vi "Fetch_DMM2831E .vi"(3 "error in (no error)":errorcluster, 5 "VISA resource name":refnum<visa-resource-name>) -> (0 "error out":errorcluster, 1 "Measurement":dbl, 2 "VISA resource name out":refnum<visa-resource-name>)   [LabVIEW 2023]
uses:
  <instrlib>/BK Precision 5491B/BK Precision 5491B.lvlib
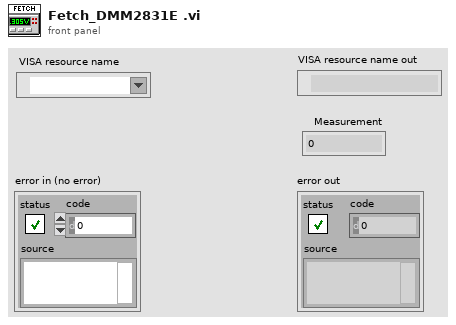
[diagram p1: front panel]
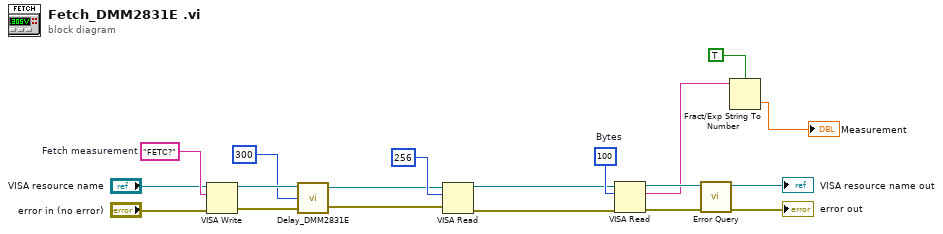
[diagram p0: block diagram]
diagram:
  w14 = "FETC?"  # Fetch measurement
  w19 = u32 100  # Bytes
  n1 = VISA Write(VISA resource name="VISA resource name", write buffer=w14, error in (no error)="error in (no error)") -> (VISA resource name out=w5:refnum<visa-resource-name>, error out=w4:errorcluster)  [unwired: 1 out]
  n2 = call "Delay_DMM2831E.vi"("error in (no error)"=w4, "Delay Time (0)"=u32 300, "Instrument In"=w5) -> ("error out"=w2:errorcluster, "Instrument Out"=w3:refnum<visa-resource-name>)
  n3 = VISA Read(VISA resource name=w3, byte count=u32 256, error in (no error)=w2) -> (VISA resource name out=w13:refnum<visa-resource-name>, error out=w12:errorcluster)  [unwired: 2 out]
  n4 = VISA Read(VISA resource name=w13, byte count=w19, error in (no error)=w12) -> (VISA resource name out=w18:refnum<visa-resource-name>, read buffer=w8:string, error out=w17:errorcluster)  [unwired: 1 out]
  n5 = call <instrlib>:"Error Query.vi"("error in (no error)"=w17, "VISA resource name"=w18) -> ("error out"=→"error out":errorcluster, "VISA resource name out"=→"VISA resource name out":refnum<visa-resource-name>)  [unwired: 7 in, 1 out]
  n6 = Fract/Exp String To Number(use system decimal point (T)=TRUE, string=w8) -> (number=→"Measurement":dbl)  [unwired: 2 in, 1 out]
